vi "maximum.vi"(10 "y":i32, 11 "x":i32) -> (3 "max":i32)   [LabVIEW 2018]
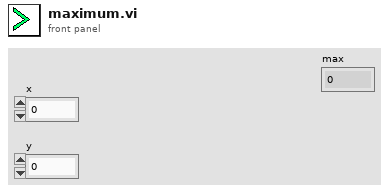
[diagram p1: front panel]
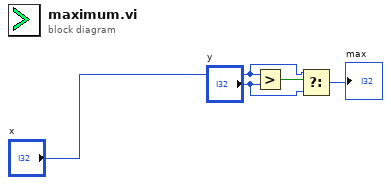
[diagram p0: block diagram]
diagram:
  n1 = Greater?(x="x", y="y") -> (0:w2:bool)
  n2 = Select(t="x", s=w2, f="y") -> (s? t:f=→"max":i32)
